vi "GetRoutes.vi"(8 "error in (no error)":errorcluster, 11 "reference in":refnum<class "Switch_Manager.lvclass">) -> (0 "error out":errorcluster, 2 "Routes":T1(array[cluster]), 3 "reference in":refnum<class "Switch_Manager.lvclass">)   [LabVIEW 2022 SP3, in "Switch_Manager.lvlib" / "Switch_Manager.lvclass"]
uses:
  Switch_Manager.lvclass
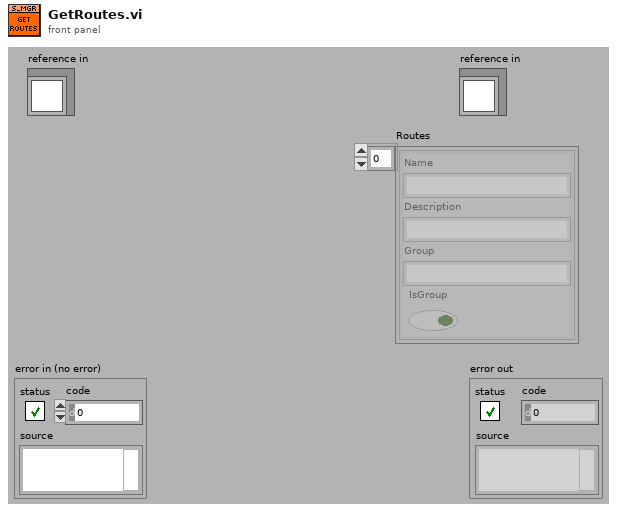
[diagram p1: front panel]
types:
  T1 = cluster{"Name":string, "Description":string, "Group":string, "IsGroup":bool}[]
  T2 = cluster{"Name":string, "Description":string, "Group":string, "IsGroup":bool}
  T3 = typedef "Switch_Manager.lvlib/Switch_Manager.lvclass/ObjectAttributes.ctl" = cluster{"Config":T4, "State":bool[], "Switches":refnum<class "SwitchBase.lvclass">[], "SwitchName":string[], "SwitchMap":T5[], "UpdateEvent":refnum<user-event>, "ParentEvent":refnum<user-event>, "Tree":bool[]}
  T4 = typedef "Switch_Manager.lvlib/Switch_Manager.lvclass/Config.ctl" = cluster{"default":string}
  T5 = typedef "Switch_Manager.lvlib/Switch_Manager.lvclass/SwitchMap.ctl" = cluster{"Name":string, "Description":string, "Group":string, "IsGroup":bool, "Switches":string[]}
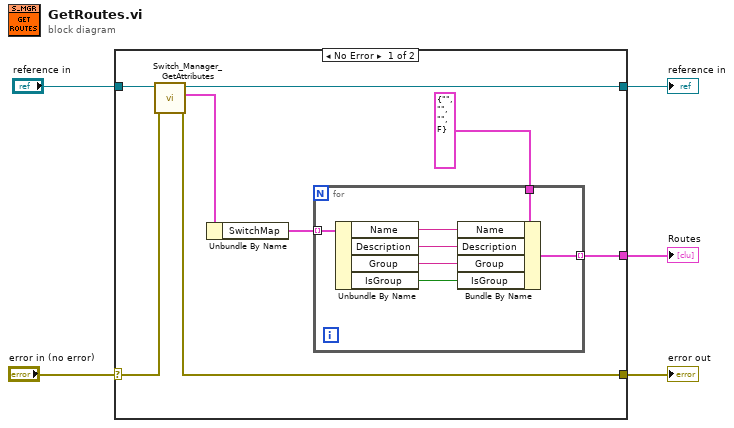
[diagram p0: block diagram]
diagram:
  n1 = case shown="No Error" "error in (no error)" {
    selector: "error in (no error)" -> [w13 w22]
    tunnel: [w11 w22] -> w4
    tunnel: [w9 w21] -> w2
    tunnel: "reference in" -> [w10 w21]
    tunnel: [w6 _] -> w1
    frame No Error {
      n2 = call "Switch_Manager_GetAttributes.vi"("error in (no error)"=w13, "reference in"=w10) -> ("error out"=w11:errorcluster, "Data"=w12:T3, "reference out"=w9:refnum<class "Switch_Manager.lvclass">)  [unwired: 6 in, 1 out]
      n3 = Unbundle By Name(w12) -> ("SwitchMap"=w7:T5[])
      n4 = for {
        tunnel: T2 {"Name"="", "Description"="", "Group"="", "IsGroup"=FALSE} ("Route") -> [w20]
        tunnel: w7 -> [w19] mode=indexing
        tunnel: [w14] -> w6 mode=indexing
        n5 = Unbundle By Name(w19) -> ("Name"=w18:string, "Description"=w17:string, "Group"=w16:string, "IsGroup"=w15:bool)
        n6 = Bundle By Name(cluster=w20, "Name"=w18, "Description"=w17, "Group"=w16, "IsGroup"=w15) -> (w14:T2)
      }
    }
    frame Error {
    }
  }
  "error out" <- w4
  "reference in" <- w2
  "Routes" <- w1
